vi "PMBus Group Cmd.vi"(5 "PEC":u8, 6 "CmdNum":u8, 7 "pGroupCmdData":u8[](array[numeric])=array[10240 elements], 9 "PMBusIndex":i32, 10 "DevIndex":i32, 11 "DevType":i32) -> (2 "function return":i32, 3 "pGroupCmdData out":u8[](array[numeric]))   [LabVIEW 2010, in "ControlPMBus.lvlib"]
doc: "int WINAPI PMBus_GroupCmd(int DevType,int DevIndex,int PMBusIndex,unsigned char *pGroupCmdData,unsigned char CmdNum,unsigned char PEC);"
uses:
  ControlPMBus.lvlib
  ControlPMBus/Ginkgo_Driver.dll
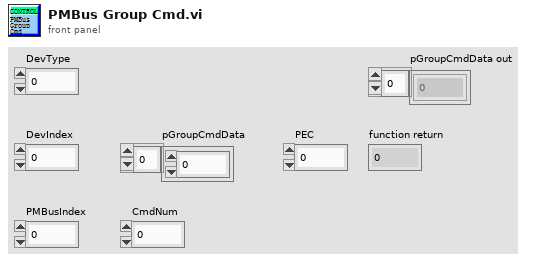
[diagram p1: front panel]
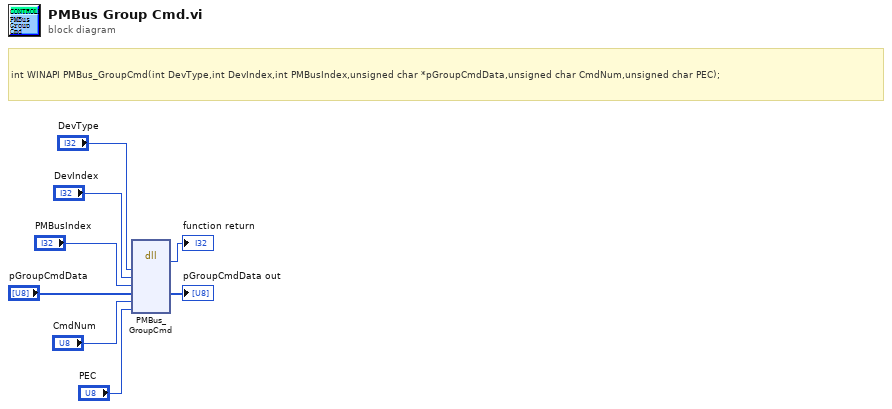
[diagram p0: block diagram]
diagram:
  # "int WINAPI PMBus_GroupCmd(int DevType,int DevIndex,int PMBusIndex,unsigned char *pGroupCmdData,unsigned char CmdNum,unsigned char PEC);"
  n1 = dll-call lib="E:/Project/vt_ginkgo/truck/Ginkgo Driver/vs2010/Ginkgo_USB-I2C&SPI&CAN_API_v2.0.3.3/lib/labview_32bit/ControlPMBus/Ginkgo_Driver.*" fn="PMBus_GroupCmd"("DevType"="DevType", "DevIndex"="DevIndex", "PMBusIndex"="PMBusIndex", "pGroupCmdData"="pGroupCmdData", "CmdNum"="CmdNum", "PEC"="PEC") -> (→"function return":i32, "pGroupCmdData"=→"pGroupCmdData out":u8[])  [unwired: 8 in, 2 out]
